vi "cam0-槽位合理角位的判断.vi"(6 "判断所在侧":bool, 8 "width":sgl, 9 "槽在中心到产品连线所在侧":enum16{"左侧-逆时针向", "右侧-顺时针向"}(ring), 10 "槽正对产品角度允许偏差以内":bool, 11 "槽指向最大允许夹角真":bool) -> (1 "属于合理情况":bool, 2 "widthOut":sgl)   [LabVIEW 2015]
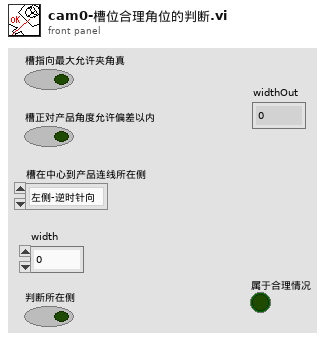
[diagram p1: front panel]
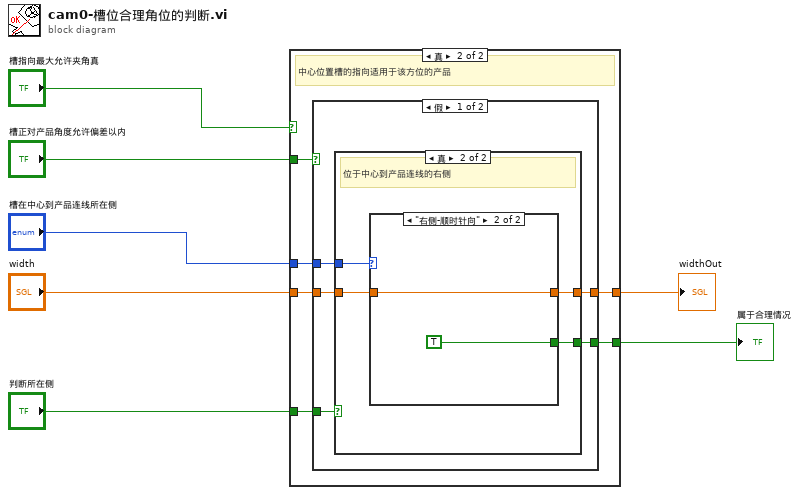
[diagram p0: block diagram]
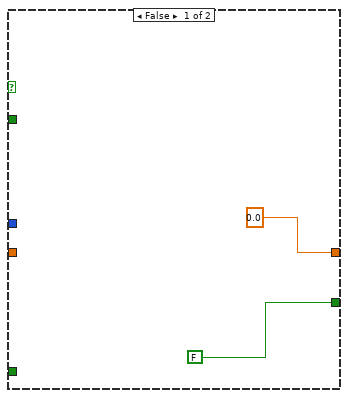
[diagram p2: hidden frame]
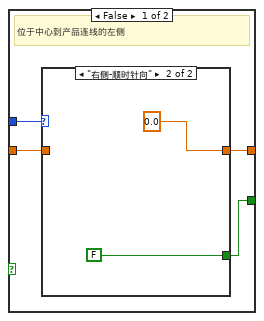
[diagram p3: hidden frame]
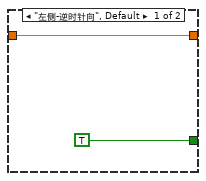
[diagram p4: hidden frame]
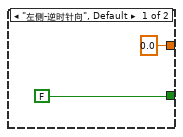
[diagram p5: hidden frame]
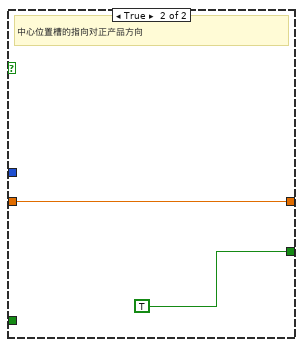
[diagram p6: hidden frame]
diagram:
  n1 = case "条件结构" shown="真" "槽指向最大允许夹角真" {
    tunnel: "判断所在侧" -> [_ w15]
    tunnel: "槽在中心到产品连线所在侧" -> [_ w14]
    tunnel: "width" -> [_ w13]
    tunnel: [FALSE w12] -> w1
    tunnel: [sgl 0.0 ("width") w11] -> w2
    tunnel: "槽正对产品角度允许偏差以内" -> [_ w10]
    frame False {
    }
    frame True {
      # "中心位置槽的指向适用于该方位的产品"
      n2 = case shown="假" w10 {
        tunnel: w15 -> [w20 _]
        tunnel: w14 -> [w19 _]
        tunnel: w13 -> [w18 w37]
        tunnel: [w17 TRUE] -> w12
        tunnel: [w16 w37] -> w11
        frame False {
          n3 = case shown="真" w20 {
            tunnel: w19 -> [w24 w32]
            tunnel: w18 -> [w23 w31]
            tunnel: [w22 w30] -> w16
            tunnel: [w21 w29] -> w17
            frame False {
              # "位于中心到产品连线的左侧"
              n4 = case shown="\"右侧-顺时针向\"" w24 {
                tunnel: [w26 sgl 0.0 ("width")] -> w22
                tunnel: w23 -> [w26 _]
                tunnel: [TRUE FALSE] -> w21
                frame "左侧-逆时针向", Default {
                }
                frame "右侧-顺时针向" {
                }
              }
            }
            frame True {
              # "位于中心到产品连线的右侧"
              n5 = case shown="\"右侧-顺时针向\"" w32 {
                tunnel: [sgl 0.0 ("width") w36] -> w30
                tunnel: w31 -> [_ w36]
                tunnel: [FALSE TRUE] -> w29
                frame "左侧-逆时针向", Default {
                }
                frame "右侧-顺时针向" {
                }
              }
            }
          }
        }
        frame True {
          # "中心位置槽的指向对正产品方向"
        }
      }
    }
  }
  "widthOut" <- w2
  "属于合理情况" <- w1
